vi "Reset Origins.vi"(8 "error in (no error)":errorcluster, 11 "VI Refnum in":refnum<vi>) -> (0 "error out":errorcluster, 3 "VI Refnum out":refnum<vi>)   [LabVIEW 2019, in "Builtins.lvlib"]
doc: "Resets all front panel panes to the 0, 0 origins.\n\nCreated by: Ryan Pacini"
uses:
  Builtins.lvlib
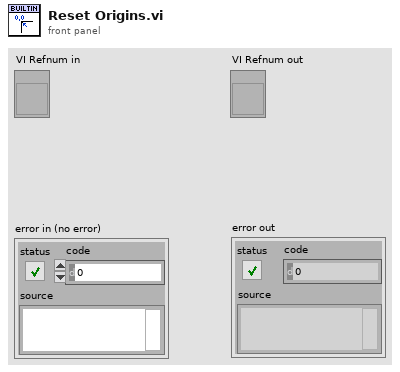
[diagram p1: front panel]
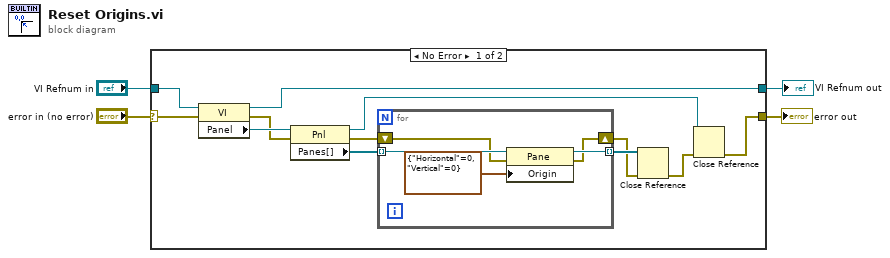
[diagram p0: block diagram]
diagram:
  n1 = case shown="No Error" "error in (no error)" {
    selector: "error in (no error)" -> [w16 w22]
    tunnel: "VI Refnum in" -> [w15 w23]
    tunnel: [w6 w23] -> w2
    tunnel: [w5 w22] -> w1
    frame No Error {
      n2 = property class="VI"(reference=w15, error in=w16) -> (reference out=w6:refnum<vi>, error out=w13:errorcluster, "Panel"=w14:refnum<vi>)
      n3 = property class="Pnl"(reference=w14, error in=w13) -> (reference out=w8:refnum<vi>, error out=w11:errorcluster, "Panes[]"=w12:refnum<vi>[])
      n4 = for {
        tunnel: w12 -> [w21] mode=indexing
        tunnel: [w18] -> w10 mode=indexing
        shift-right: [w17] -> w9
        shift-left: w11 -> [w20]
        n5 = property class="Pane"(reference=w21, error in=w20, "Origin"=cluster{"Horizontal":i16, "Vertical":i16} {"Horizontal"=0, "Vertical"=0}) -> (reference out=w18:refnum<vi>, error out=w17:errorcluster)
      }
      n6 = Close Reference(reference=w10, error in (no error)=w9) -> (error out=w7:errorcluster)
      n7 = Close Reference(reference=w8, error in (no error)=w7) -> (error out=w5:errorcluster)
    }
    frame Error {
    }
  }
  "VI Refnum out" <- w2
  "error out" <- w1
